vi "Where XYZ.vi"(0 "ASI stage":T1, 5 "stop if out of range":bool, 11 "error in (no error)":errorcluster) -> (4 "location":cluster{"X out":dbl, "Y out":dbl, "Z out":dbl} {"Z out" format="%#.4f"; "Y out" format="%#.4f"; "X out" format="%#.4f"}, 6 "out of range":bool, 15 "error out":errorcluster)   [LabVIEW 2010]
uses:
  stage properties.ctl
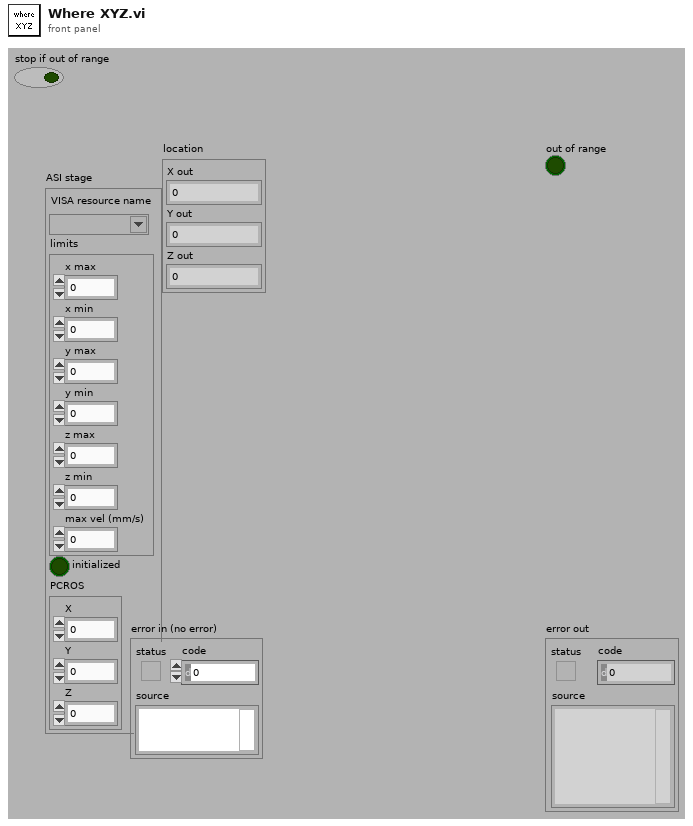
[diagram p1: front panel]
types:
  T1 = typedef "stage properties.ctl" = cluster{"VISA resource name":refnum<visa-resource-name>, "limits":cluster{"x max":dbl, "x min":dbl, "y max":dbl, "y min":dbl, "z max":dbl, "z min":dbl, "max vel (mm/s)":dbl}, "initialized":bool, "PCROS":cluster{"X":dbl, "Y":dbl, "Z":dbl}}
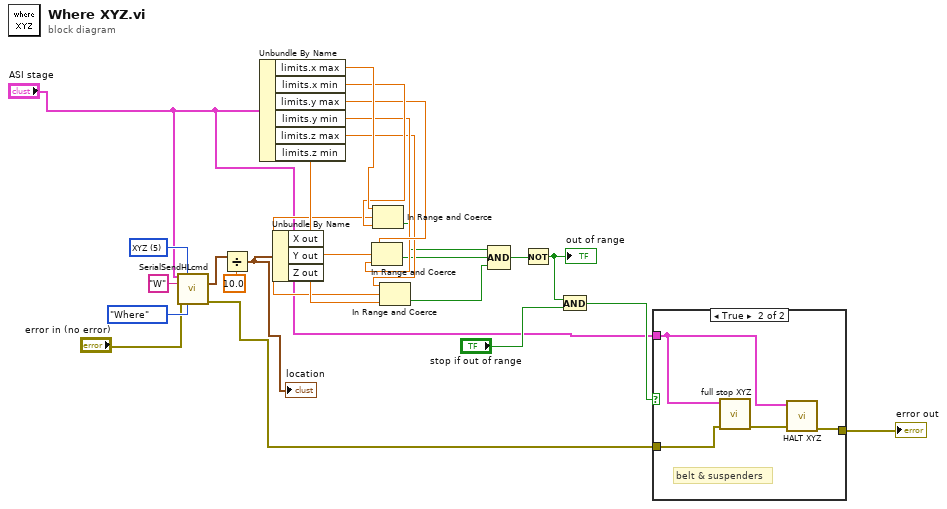
[diagram p0: block diagram]
diagram:
  w26 = u16 5 items=["No axis", "X", "Y", "Z", "XY", "XYZ"] ("Axis configuration")
  n1 = call "SerialSendHLcmd.vi"("ASI stage"="ASI stage", "Axis configuration"=w26, "Command"="W", "error in (no error)"="error in (no error)", "Command type"=enum16{"Query", "Where", "Imperative", "DU Y"}."Where") -> ("data out"=w9:cluster{"X out":dbl, "Y out":dbl, "Z out":dbl}, "error out"=w5:errorcluster)  [unwired: 8 in, 1 out]
  n2 = Divide(x=w9, y=10.0) -> (x/y=w1:cluster{"X out":dbl, "Y out":dbl, "Z out":dbl})
  "location" <- w1
  n3 = Unbundle By Name("ASI stage") -> ("limits.x max"=w22:dbl, "limits.x min"=w21:dbl, "limits.y max"=w20:dbl, "limits.y min"=w19:dbl, "limits.z max"=w18:dbl, "limits.z min"=w17:dbl)
  n4 = Unbundle By Name(w1) -> ("X out"=w16:dbl, "Y out"=w15:dbl, "Z out"=w14:dbl)
  n5 = In Range and Coerce(upper limit=w20, x=w15, lower limit=w19) -> (In Range?=w12:bool)  [unwired: 1 out]
  n6 = In Range and Coerce(upper limit=w22, x=w16, lower limit=w21) -> (In Range?=w13:bool)  [unwired: 1 out]
  n7 = In Range and Coerce(upper limit=w18, x=w14, lower limit=w17) -> (In Range?=w11:bool)  [unwired: 1 out]
  n8 = Compound Arithmetic op=AND(w13, w12, w11) -> (w10:bool)
  n9 = Not(x=w10) -> (.not. x?=w8:bool)
  "out of range" <- w8
  n10 = And(x=w8, y="stop if out of range") -> (x .and. y?=w6:bool)
  n11 = case shown="True" w6 {
    tunnel: "ASI stage" -> [_ w30]
    tunnel: w5 -> [w27 w29]
    tunnel: [w27 w31] -> w4
    frame False {
    }
    frame True {
      # "belt & suspenders"
      n12 = call "full stop XYZ.vi"("error in (no error)"=w29, "ASI stage"=w30) -> ("error out"=w28:errorcluster)  [unwired: 9 in]
      n13 = call "HALT XYZ.vi"("error in (no error)"=w28, "ASI stage"=w30) -> ("error out"=w31:errorcluster)  [unwired: 9 in]
    }
  }
  "error out" <- w4
